vi "PI Stabilization.vi"() -> ()   [LabVIEW 2010]
uses:
  Global Variables/Global Stop.vi
panel:
  in  "Proportional Correction Factor":dbl=300.0
  in  "Activate Output":bool
  in  "Integration Time Interval":dbl=200.0
  in  "Reset Integral":bool
  out "Thick Etalon Pos Setp on Activation":i32
  out "Wavenumber on Activation":dbl format="%.4f"
  in  "Correction Output":bool
  out "correction steps":dbl
  in  "Difference Threshold":dbl=0.05
  in  "Integral Correction Factor":dbl=0.005
  out "New Wavemeter Value":bool
  out "Out of Range":bool
  in  "Stop":bool
  out "PStab loop counter":i32
  in  "Thick Etalon Position Setpoint":i32
  in  "Invert Output":bool=TRUE
  in  "Wavenumber Setpoint":dbl format="%.4f"
  out "WS7 Ch1 Wavenumber":dbl format="%.4f"
  # "Invert Output\nif moving beyond\nFlash Position"
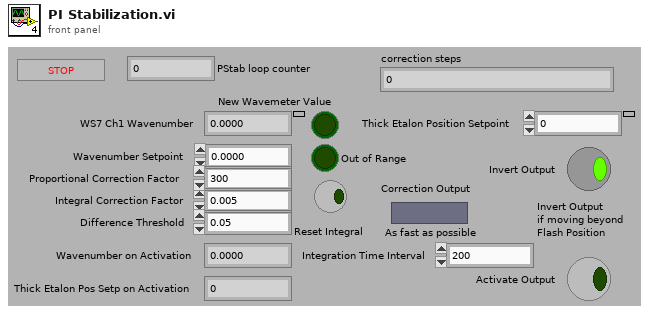
[diagram p1: front panel]
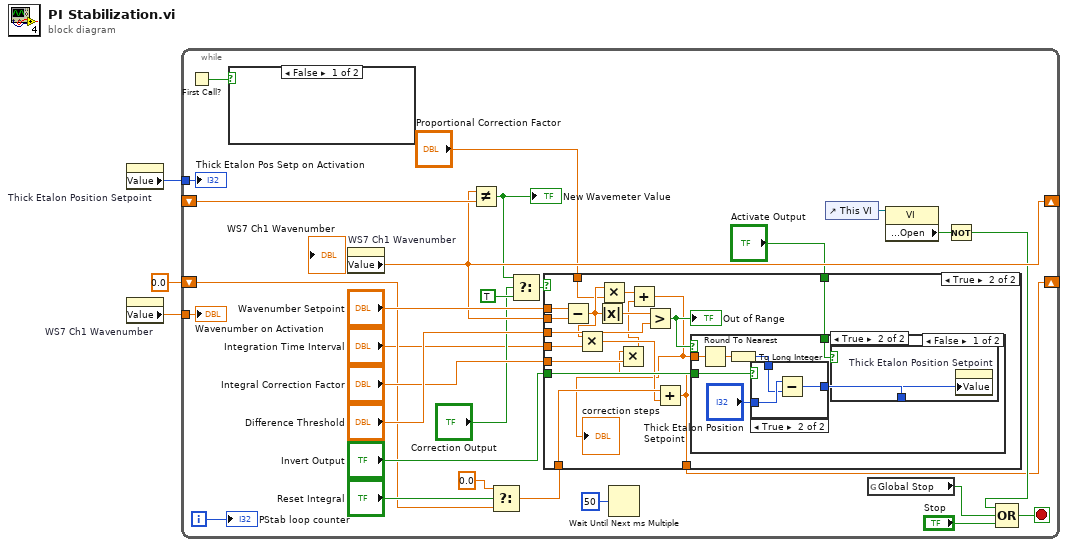
[diagram p0: block diagram]
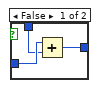
[diagram p4: hidden frame]
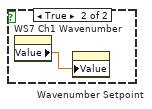
[diagram p6: hidden frame]
diagram:
  n1 = property on="Thick Etalon Position Setpoint" class="DigNum (strict)"() -> ("Value"=w2:i32)  [unwired: 2 in, 2 out]
  n2 = property on="WS7 Ch1 Wavenumber" class="DigNum (strict)"() -> ("Value"=w3:dbl)  [unwired: 2 in, 2 out]
  n3 = while {
    shift-right: [w29] -> _
    shift-left: _ -> [w31]
    tunnel: w3 -> [w13]
    tunnel: w2 -> [w12]
    shift-right: [w6] -> _
    shift-left: 0.0 -> [w9]
    i -> [w27]
    stop <- w17 stop-if-true
    n4 = First Call?() -> (First Call?: T/F=w32:bool)
    n5 = case shown="False" w32 {
      frame False {
      }
      frame True {
        n6 = property on="WS7 Ch1 Wavenumber" class="DigNum (strict)"() -> ("Value"=w65:dbl)  [unwired: 2 in, 2 out]
        n7 = property on="Wavenumber Setpoint" class="DigNum (strict)"("Value"=w65) -> ()  [unwired: 2 in, 2 out]
      }
    }
    n8 = property on="WS7 Ch1 Wavenumber" class="DigNum (strict)"() -> ("Value"=w29:dbl)  [unwired: 2 in, 2 out]
    n9 = Not Equal?(x=w29, y=w31) -> (x != y?=w22:bool)
    "New Wavemeter Value" <- w22
    n10 = Select(t=0.0, s="Reset Integral", f=w9) -> (s? t:f=w7:dbl)
    n11 = Select(t=w22, s="Correction Output", f=TRUE) -> (s? t:f=w23:bool)
    n12 = case shown="True" w23 {
      tunnel: "Wavenumber Setpoint" -> [_ w50]
      tunnel: w29 -> [_ w49]
      tunnel: "Difference Threshold" -> [_ w46]
      tunnel: "Integral Correction Factor" -> [_ w45]
      tunnel: "Invert Output" -> [_ w44]
      tunnel: "Integration Time Interval" -> [_ w43]
      tunnel: w7 -> [w33 w42]
      tunnel: [w33 w40] -> w6
      tunnel: "Activate Output" -> [_ w39]
      tunnel: "Proportional Correction Factor" -> [_ w37]
      frame False {
      }
      frame True {
        n13 = Subtract(x=w50, y=w49) -> (x-y=w38:dbl)
        n14 = Multiply(x=w38, y=w43) -> (x*y=w41:dbl)
        n15 = Absolute Value(x=w38) -> (abs(x)=w48:dbl)
        n16 = Multiply(x=w38, y=w37) -> (x*y=w36:dbl)
        n17 = Greater?(x=w48, y=w46) -> (0:w47:bool)
        "Out of Range" <- w47
        n18 = Add(x=w42, y=w41) -> (x+y=w40:dbl)
        n19 = Multiply(x=w40, y=w45) -> (x*y=w34:dbl)
        n20 = Add(x=w36, y=w34) -> (x+y=w35:dbl)
        "correction steps" <- w35
        n21 = case shown="False" w47 {
          tunnel: w44 -> [w55 _]
          tunnel: w39 -> [w52 _]
          tunnel: w35 -> [w51 _]
          frame False {
            n22 = Round To Nearest(number=w51) -> (nearest integer value=w54:dbl)
            n23 = To Long Integer(number=w54) -> (32bit integer=w53:i32)
            n24 = case shown="True" w55 {
              tunnel: "Thick Etalon Position Setpoint" -> [w61 w64]
              tunnel: w53 -> [w60 w63]
              tunnel: [w59 w62] -> w56
              frame False {
                n25 = Add(x=w61, y=w60) -> (x+y=w59:i32)
              }
              frame True {
                n26 = Subtract(x=w64, y=w63) -> (x-y=w62:i32)
              }
            }
            n27 = case shown="True" w52 {
              tunnel: w56 -> [_ w58]
              frame False {
              }
              frame True {
                n28 = property on="Thick Etalon Position Setpoint" class="DigNum (strict)"("Value"=w58) -> ()  [unwired: 2 in, 2 out]
              }
            }
          }
          frame True {
          }
        }
      }
    }
    n29 = Wait Until Next ms Multiple(millisecond multiple=u32 50) -> ()  [unwired: 1 out]
    n30 = control-ref of="This VI"() -> (w18:refnum<vi>)
    n31 = global read "Global Stop.vi" "Global Stop"() -> (w15:bool)
    n32 = property class="VI"(reference=w18) -> ("Front Panel.Open"=w19:bool)  [unwired: 1 in, 2 out]
    n33 = Not(x=w19) -> (.not. x?=w16:bool)
    n34 = Compound Arithmetic op=OR(w16, w15, "Stop") -> (w17:bool)
    "PStab loop counter" <- w27
    "Wavenumber on Activation" <- w13
    "Thick Etalon Pos Setp on Activation" <- w12
  }
